vi "Launch.vi"(8 "error in (no error)":errorcluster, 10 "Show Front Panel? (F)":bool, 11 "API-Reference in":refnum<data-value>) -> (0 "error out":errorcluster, 1 "Already Launched":bool, 3 "API-Reference out":refnum<data-value>)   [LabVIEW 2018, in "Scripting.lvlib" / "Actor.lvclass"]
uses:
  Actor.lvclass
  API-Data.ctl
  Front-Panel State.ctl
  Did Stop.ctl
  All-Enqueuers.ctl
  Broadcast Enqueuers.ctl
  Did Initialize.ctl
  Request-Enqueuers.ctl
  Get State.ctl
  State.ctl
  Stop.ctl
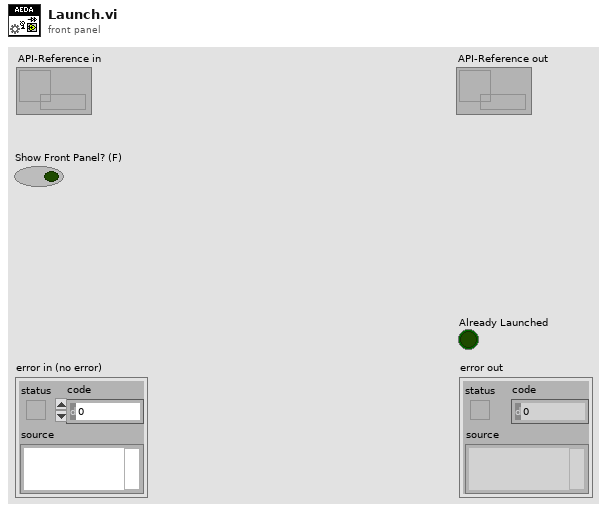
[diagram p1: front panel]
types:
  T1 = typedef "Scripting.lvlib/Actor.lvclass/Front-Panel State.ctl" = enum16{"Don't Show", "Show"}
  T2 = typedef "Scripting.lvlib/Actor.lvclass/API-Data.ctl" = cluster{"Launch":refnum<notifier>, "Did Stop Message":refnum<event-registration>, "Did Stop Enqueuer":refnum<user-event>, "Enqueuers":T3}
  T3 = typedef "Scripting.lvlib/Actor.lvclass/All-Enqueuers.ctl" = cluster{"Broadcasts":T4, "Requests":T5}
  T4 = typedef "Scripting.lvlib/Actor.lvclass/Broadcast Enqueuers.ctl" = cluster{"Did Initialize":refnum<user-event>}
  T5 = typedef "Scripting.lvlib/Actor.lvclass/Request-Enqueuers.ctl" = cluster{"Get State":refnum<user-event>, "Stop":refnum<user-event>}
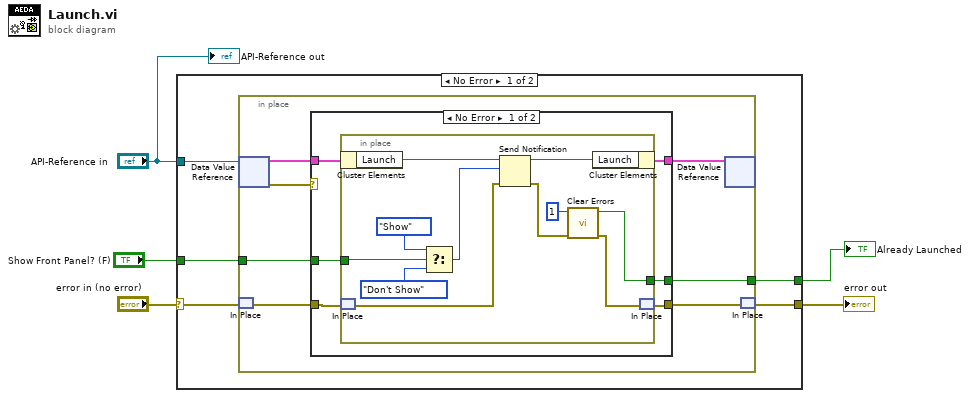
[diagram p0: block diagram]
diagram:
  n1 = case shown="No Error" "error in (no error)" {
    selector: "error in (no error)" -> [w10 w37]
    tunnel: [w9 w37] -> w4
    tunnel: "API-Reference in" -> [w6 _]
    tunnel: [w8 _] -> w3
    tunnel: "Show Front Panel? (F)" -> [w7 _]
    frame No Error {
      n2 = in-place {
        in-place-border: [w12] -> w8
        in-place-border: w7 -> [w11]
        n3 = in-place-dvr #1(w6) -> (w16:T2, w17:errorcluster)
        n4 = in-place-match #2(w10) -> (w14:errorcluster)
        n5 = case shown="No Error" w17 {
          selector: w17 -> [_ w36]
          tunnel: w16 -> [w19 w35]
          tunnel: [w18 w35] -> w15
          tunnel: w14 -> [w23 _]
          tunnel: [w22 w36] -> w13
          tunnel: [w21 _] -> w12
          tunnel: w11 -> [w20 _]
          frame No Error {
            n6 = in-place {
              in-place-border: [w31] -> w21
              in-place-border: w20 -> [w27]
              n7 = in-place-cluster #3(w19) -> ("Launch"=w30:refnum<notifier>)
              n8 = in-place-match #4(w23) -> (w34:errorcluster)
              n9 = Select(t=Front-Panel_State."Show" ("notification"), s=w27, f=Front-Panel_State."Don't Show" ("notification")) -> (s? t:f=w24:T1)
              n10 = Send Notification(notification=w24, notifier=w30, error in (no error)=w34) -> (notifier out=w33:refnum<notifier>, error out=w29:errorcluster)
              n11 = call <vilib>:"Clear Errors.vi"("error in (no error)"=w29, "specific error code to clear (0: all)"=1) -> ("error out"=w28:errorcluster, "specific error cleared?"=w31:bool)  [unwired: 4 in]
              n12 = in-place-cluster #3("Launch"=w33) -> (w18:T2)
              n13 = in-place-match #4(w28) -> (w22:errorcluster)
            }
          }
          frame Error {
          }
        }
        n14 = in-place-dvr #1(w15) -> ()  [unwired: 2 out]
        n15 = in-place-match #2(w13) -> (w9:errorcluster)
      }
    }
    frame Error {
    }
  }
  "error out" <- w4
  "Already Launched" <- w3
  "API-Reference out" <- "API-Reference in"
